vi "calculate_orientation_xyz.vi"(5 "orientation YPR":cluster{"yaw":dbl, "pitch":dbl, "roll":dbl}) -> (2 "pose":dbl[](array[numeric]))   [LabVIEW 2019, in "Lib_Simx.lvlib"]
doc: "Converts orientation Yaw, Pitch and roll to X,Y,Z,W ."
uses:
  Lib_Simx.lvlib
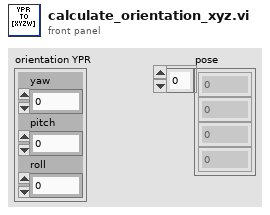
[diagram p1: front panel]
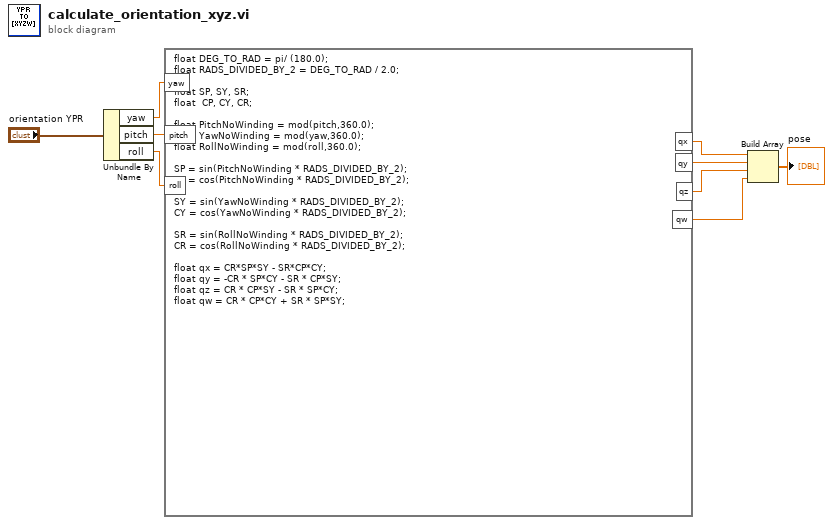
[diagram p0: block diagram]
diagram:
  n1 = Unbundle By Name("orientation YPR") -> ("yaw"=w8:dbl, "pitch"=w7:dbl, "roll"=w6:dbl)
  n2 = formula code="float DEG_TO_RAD = pi/ (180.0);\nfloat RADS_DIVIDED_BY_2 = DEG_TO_RAD / 2.0;\n\nfloat SP, SY, SR;\nfloat  CP, CY, CR;\n\nfloat PitchNoWinding = mod(pitch,360.0);\nfloat YawNoWinding = mod(yaw,360.0);\nfloat RollNoWinding = mod(roll,360.0);\n\nSP = sin(PitchNoWinding * RADS_DIVIDED_BY_2);\nCP = cos(PitchNoWinding * RADS_DIVIDED_BY_2);\n\nSY = sin(YawNoWinding * RADS_DIVIDED_BY_2);\nCY = cos(YawNoWinding * RADS_DIVIDED_BY_2);\n\nSR = sin(RollNoWinding * RADS_DIVIDED_BY_2);\nCR = cos(RollNoWinding * RADS_DIVIDED_BY_2);\n\nfloat qx = CR*SP*SY - SR*CP*CY;\nfloat qy = -CR * SP*CY - SR * CP*SY;\nfloat qz = CR * CP*SY - SR * SP*CY;\nfloat qw = CR * CP*CY + SR * SP*SY;"("yaw"=w8, "pitch"=w7, "roll"=w6) -> ("qw"=w2:dbl, "qx"=w5:dbl, "qy"=w4:dbl, "qz"=w3:dbl)
  n3 = Build Array(w5, w4, w3, w2) -> (→"pose":dbl[])
